vi "ReadConfigKeys(Int32).vi"(0 "GRMActor in":refnum<class "GRMActor.lvclass">, 5 "Config Refnum":T1, 7 "Keys":string[](array[string]), 9 "Default":i32[](array[numeric]), 11 "error in (no error)":errorcluster) -> (4 "GRMActor out":refnum<class "GRMActor.lvclass">, 15 "error out":errorcluster)   [LabVIEW 2020, in "GRMActor.lvlib" / "GRMActor.lvclass"]
uses:
  GRMActor.lvclass
  <vilib>/Utility/config.llb/Config Data RefNum.ctl
  <vilib>/Utility/config.llb/Read Key (I32).vi
  <vilib>/Utility/config.llb/Write Key (I32).vi
  <vilib>/Utility/config.llb/NI_LVConfig.lvlib
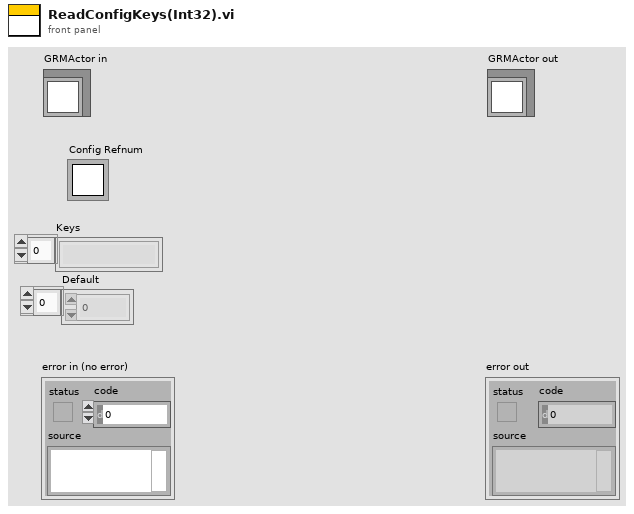
[diagram p1: front panel]
types:
  T1 = typedef "NI_LVConfig.lvlib/Config Data RefNum.ctl" = refnum<k1>
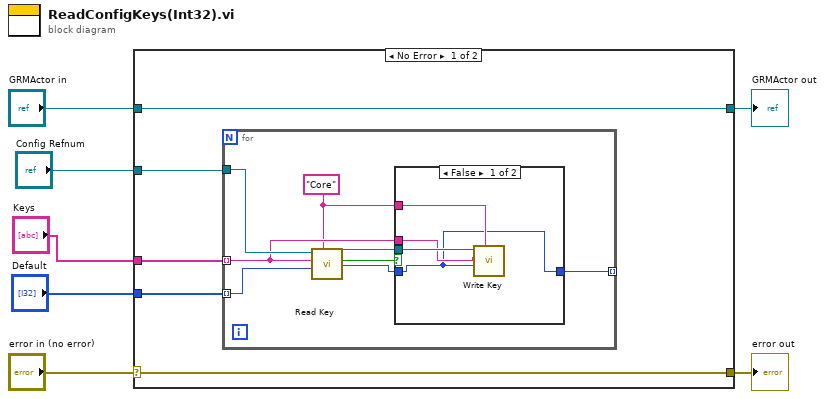
[diagram p0: block diagram]
diagram:
  n1 = case shown="No Error" "error in (no error)" {
    selector: "error in (no error)" -> [w11 w27]
    tunnel: [w11 w27] -> w6
    tunnel: [w12 w26] -> w4
    tunnel: "GRMActor in" -> [w12 w26]
    tunnel: "Config Refnum" -> [w10 _]
    tunnel: "Keys" -> [w9 _]
    tunnel: "Default" -> [w8 _]
    frame No Error {
      n2 = for {
        tunnel: w9 -> [w16] mode=indexing
        tunnel: w10 -> [w19]
        tunnel: w8 -> [w20] mode=indexing
        tunnel: [w13] -> _ mode=indexing
        w14 = "Core" ("section")
        n3 = call-poly <vilib>:"Read Key.vi"("section"=w14, "default value"=w20, "key"=w16, "refnum"=w19) -> ("value"=w15:i32, "found?"=w18:bool, "refnum out"=w17:T1)  [unwired: 4 in, 1 out]
        n4 = case shown="False" w18 {
          tunnel: w17 -> [w24 _]
          tunnel: w16 -> [w23 _]
          tunnel: w15 -> [w21 w25]
          tunnel: w14 -> [w22 _]
          tunnel: [w21 w25] -> w13
          frame False {
            n5 = call-poly <vilib>:"Write Key.vi"("section"=w22, "value"=w21, "key"=w23, "refnum"=w24) -> ()  [unwired: 5 in, 3 out]
          }
          frame True {
          }
        }
      }
    }
    frame Error {
    }
  }
  "error out" <- w6
  "GRMActor out" <- w4
